vi "sumQTY.vi"() -> ()   [LabVIEW 2012]
uses:
  <vilib>/addons/database/Connection.llb/DB Tools Open Connec (Path).vi
  <vilib>/addons/database/_DB Variant To Data/Database Variant To Data.xnode
  <vilib>/addons/database/NI_Database_API.lvlib
panel:
  out "sum 2":i32
  out "sum":i32
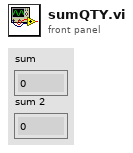
[diagram p1: front panel]
types:
  T1 = typedef "NI_Database_API.lvlib/Conn ObjectReference.ctl" = refnum<k1>
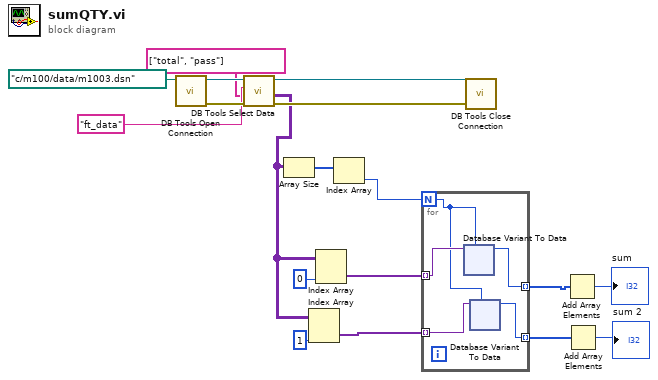
[diagram p0: block diagram]
diagram:
  n1 = call-poly <vilib>:"DB Tools Open Connection.vi"("connection information"=path "c:/m100/data/m1003.dsn") -> ("error out"=w16:errorcluster, "connection reference"=w17:T1)  [unwired: 7 in]
  n2 = call <vilib>:"DB Tools Select Data.vi"("error in (no error)"=w16, "columns"=string[] ["total", "pass"], "table"="ft_data", "connection reference"=w17) -> ("error out"=w14:errorcluster, "data"=w2:variant[][], "connection reference out"=w15:T1)  [unwired: 2 in]
  n3 = Array Size(array=w2) -> (size(s)=w11:i32[])
  n4 = Index Array(array=w2, index (col)=1) -> (element=w1:variant[])  [unwired: 1 in]
  n5 = Index Array(array=w2, index (col)=0 ("disabled index (col)")) -> (element=w9:variant[])  [unwired: 1 in]
  n6 = Index Array(array=w11) -> (element=w10:i32)  [unwired: 1 in]
  n7 = for {
    N: w10 -> [w19]
    tunnel: w9 -> [w23] mode=indexing
    tunnel: [w22] -> w7 mode=indexing
    tunnel: w1 -> [w21] mode=indexing
    tunnel: [w20] -> w5 mode=indexing
    n8 = xnode "Database Variant To Data"("database variant"=w23, "type"=w19) -> ("data"=w22:i32)  [unwired: 1 in, 1 out]
    n9 = xnode "Database Variant To Data"("database variant"=w21, "type"=w19) -> ("data"=w20:i32)  [unwired: 1 in, 1 out]
  }
  n10 = call <vilib>:"DB Tools Close Connection.vi"("error in (no error)"=w14, "connection reference"=w15) -> ()  [unwired: 5 in, 1 out]
  n11 = Add Array Elements(numeric array=w7) -> (sum=→"sum":i32)
  n12 = Add Array Elements(numeric array=w5) -> (sum=→"sum 2":i32)
